vi "Test.vi"(5 "Einheit in":string) -> (2 "Spalten Titel mit Einheiten out":string[](array[string]), 3 "LIN Ausgabetabelle  2":T1 caption="LIN Ausgabetabelle")   [LabVIEW 2020, in "EPA 1065.lvlib" / "HovaCAL Interference verificaton.lvlib"]
uses:
  HovaCAL Interference verificaton.lvlib
  Tabelle.ctl
  Linearisierung V2/Linearisierung v2.lvlib
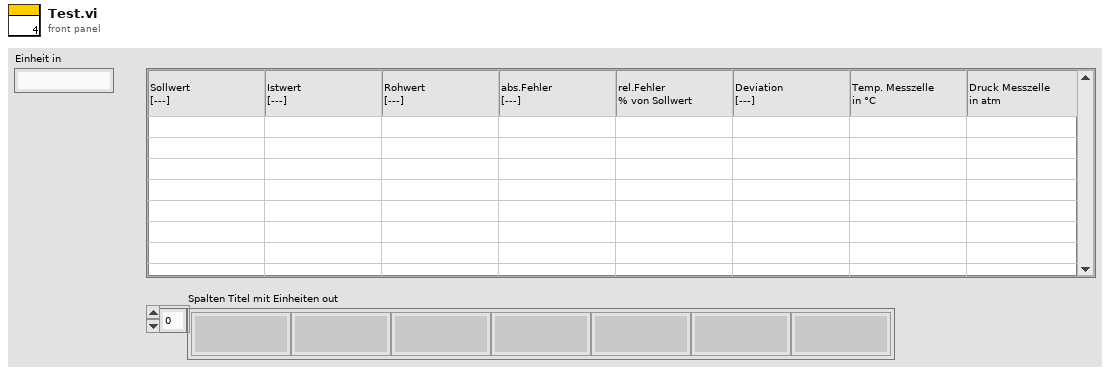
[diagram p1: front panel]
types:
  T1 = typedef "EPA 1065.lvlib/HovaCAL Interference verificaton.lvlib/Tabelle.ctl" = string[][]
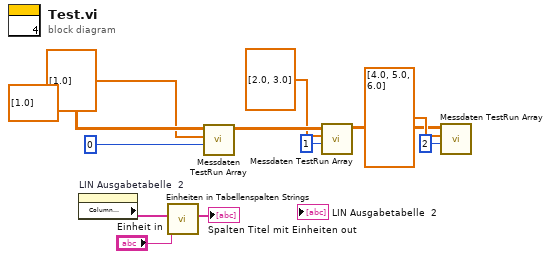
[diagram p0: block diagram]
diagram:
  n1 = property on="LIN Ausgabetabelle  2" class="Tbl (strikt)"() -> ("Column Headers[]"=w3:string[])  [unwired: 2 in, 2 out]
  n2 = call "Einheiten in Tabellenspalten Strings.vi"("Spalten Titel mit Einheiten in"=w3, "Einheit in"="Einheit in") -> ("Spalten Titel mit Einheiten out"=→"Spalten Titel mit Einheiten out":string[])  [unwired: 7 in, 2 out]
  n3 = call "Messdaten TestRun Array.vi"("Index"=0, "Array (Eingang)"=sgl[] [1.0] ("Numerisch"), "Array gesamt (Eingang)"=sgl[][] [[1.0]] ("Numerisch")) -> ("Array gesamt (Ausgang)"=w10:sgl[][])  [unwired: 4 in, 4 out]
  n4 = call "Messdaten TestRun Array.vi"("Index"=1, "Array (Eingang)"=sgl[] [2.0, 3.0] ("Array"), "Array gesamt (Eingang)"=w10) -> ("Array gesamt (Ausgang)"=w4:sgl[][])  [unwired: 4 in, 4 out]
  n5 = call "Messdaten TestRun Array.vi"("Index"=2, "Array (Eingang)"=sgl[] [4.0, 5.0, 6.0] ("Array"), "Array gesamt (Eingang)"=w4) -> ()  [unwired: 4 in, 5 out]
